vi "Teleop.vi"(10 "Match Info":T1={"Autonomous Elapsed Seconds"=0.0, "TeleOp Elapsed Seconds"=0.0, "Disabled Elapsed Seconds"=0.0, "Visited Autonomous"=FALSE, "Visited TeleOp"=FALSE, "Visited Disabled"=FALSE, "Autonomous Settings"={"Autonomous Style"=enum."Independent", "VI Refnum"=refnum}}, 11 "Call Context":T2) -> ()   [LabVIEW 2020]
doc: "This VI is called for each TeleOp packet received from the DS where the robot is not disabled. It is often used to read from the joysticks and update I/O or to update setpoints for timed control loops. It should complete and return within 20 milliseconds or it may miss DS packets."
uses:
  <vilib>/Rock Robotics/WPI/DriverStation/WPI_DriverStationDerivedRobotMode.ctl
  <vilib>/Rock Robotics/WPI/DriverStation/WPI_DriverStationMatch Info.ctl
  <vilib>/Rock Robotics/WPI/Solenoid/WPI_SolenoidValue.ctl
  <vilib>/Rock Robotics/WPI/ThirdParty/Phoenix-LabVIEW/Motor Controller/Controls/CTRE_Phoenix_MotorControl_ControlMode.ctl
  <vilib>/Rock Robotics/WPI/Utilities/WPI_GetSetVariantRefNum.vi
  <vilib>/Rock Robotics/Network Tables/NT Write Boolean Array.vi
  <vilib>/Rock Robotics/Network Tables/NT Write Numeric Array.vi
  <vilib>/Rock Robotics/Network Tables/NT Read Boolean.vi
  <vilib>/Rock Robotics/Network Tables/NT Read Number.vi
  <vilib>/Rock Robotics/WPI/Solenoid/Deprecated/WPI_SolenoidSetBool.vi
  <vilib>/Rock Robotics/Network Tables/NT Write Number.vi
  <vilib>/Rock Robotics/WPI/Solenoid/WPI_SolenoidSetEnum.vi
  Robot Global Data.vi
  <vilib>/Rock Robotics/WPI/Solenoid/Deprecated/WPI_SolenoidGetBool.vi
panel:
  out "TargetValid 5":bool
  out "TargetValid 4":bool
  out "POVs":i16[](array[numeric])
  out "Sample Slider 0":dbl(slide) scale=0.0..5.0
  out "Sample Boolean 1":bool
  out "Sample Boolean 0":bool
  # "April tags"
  # "Retroreflective tape"
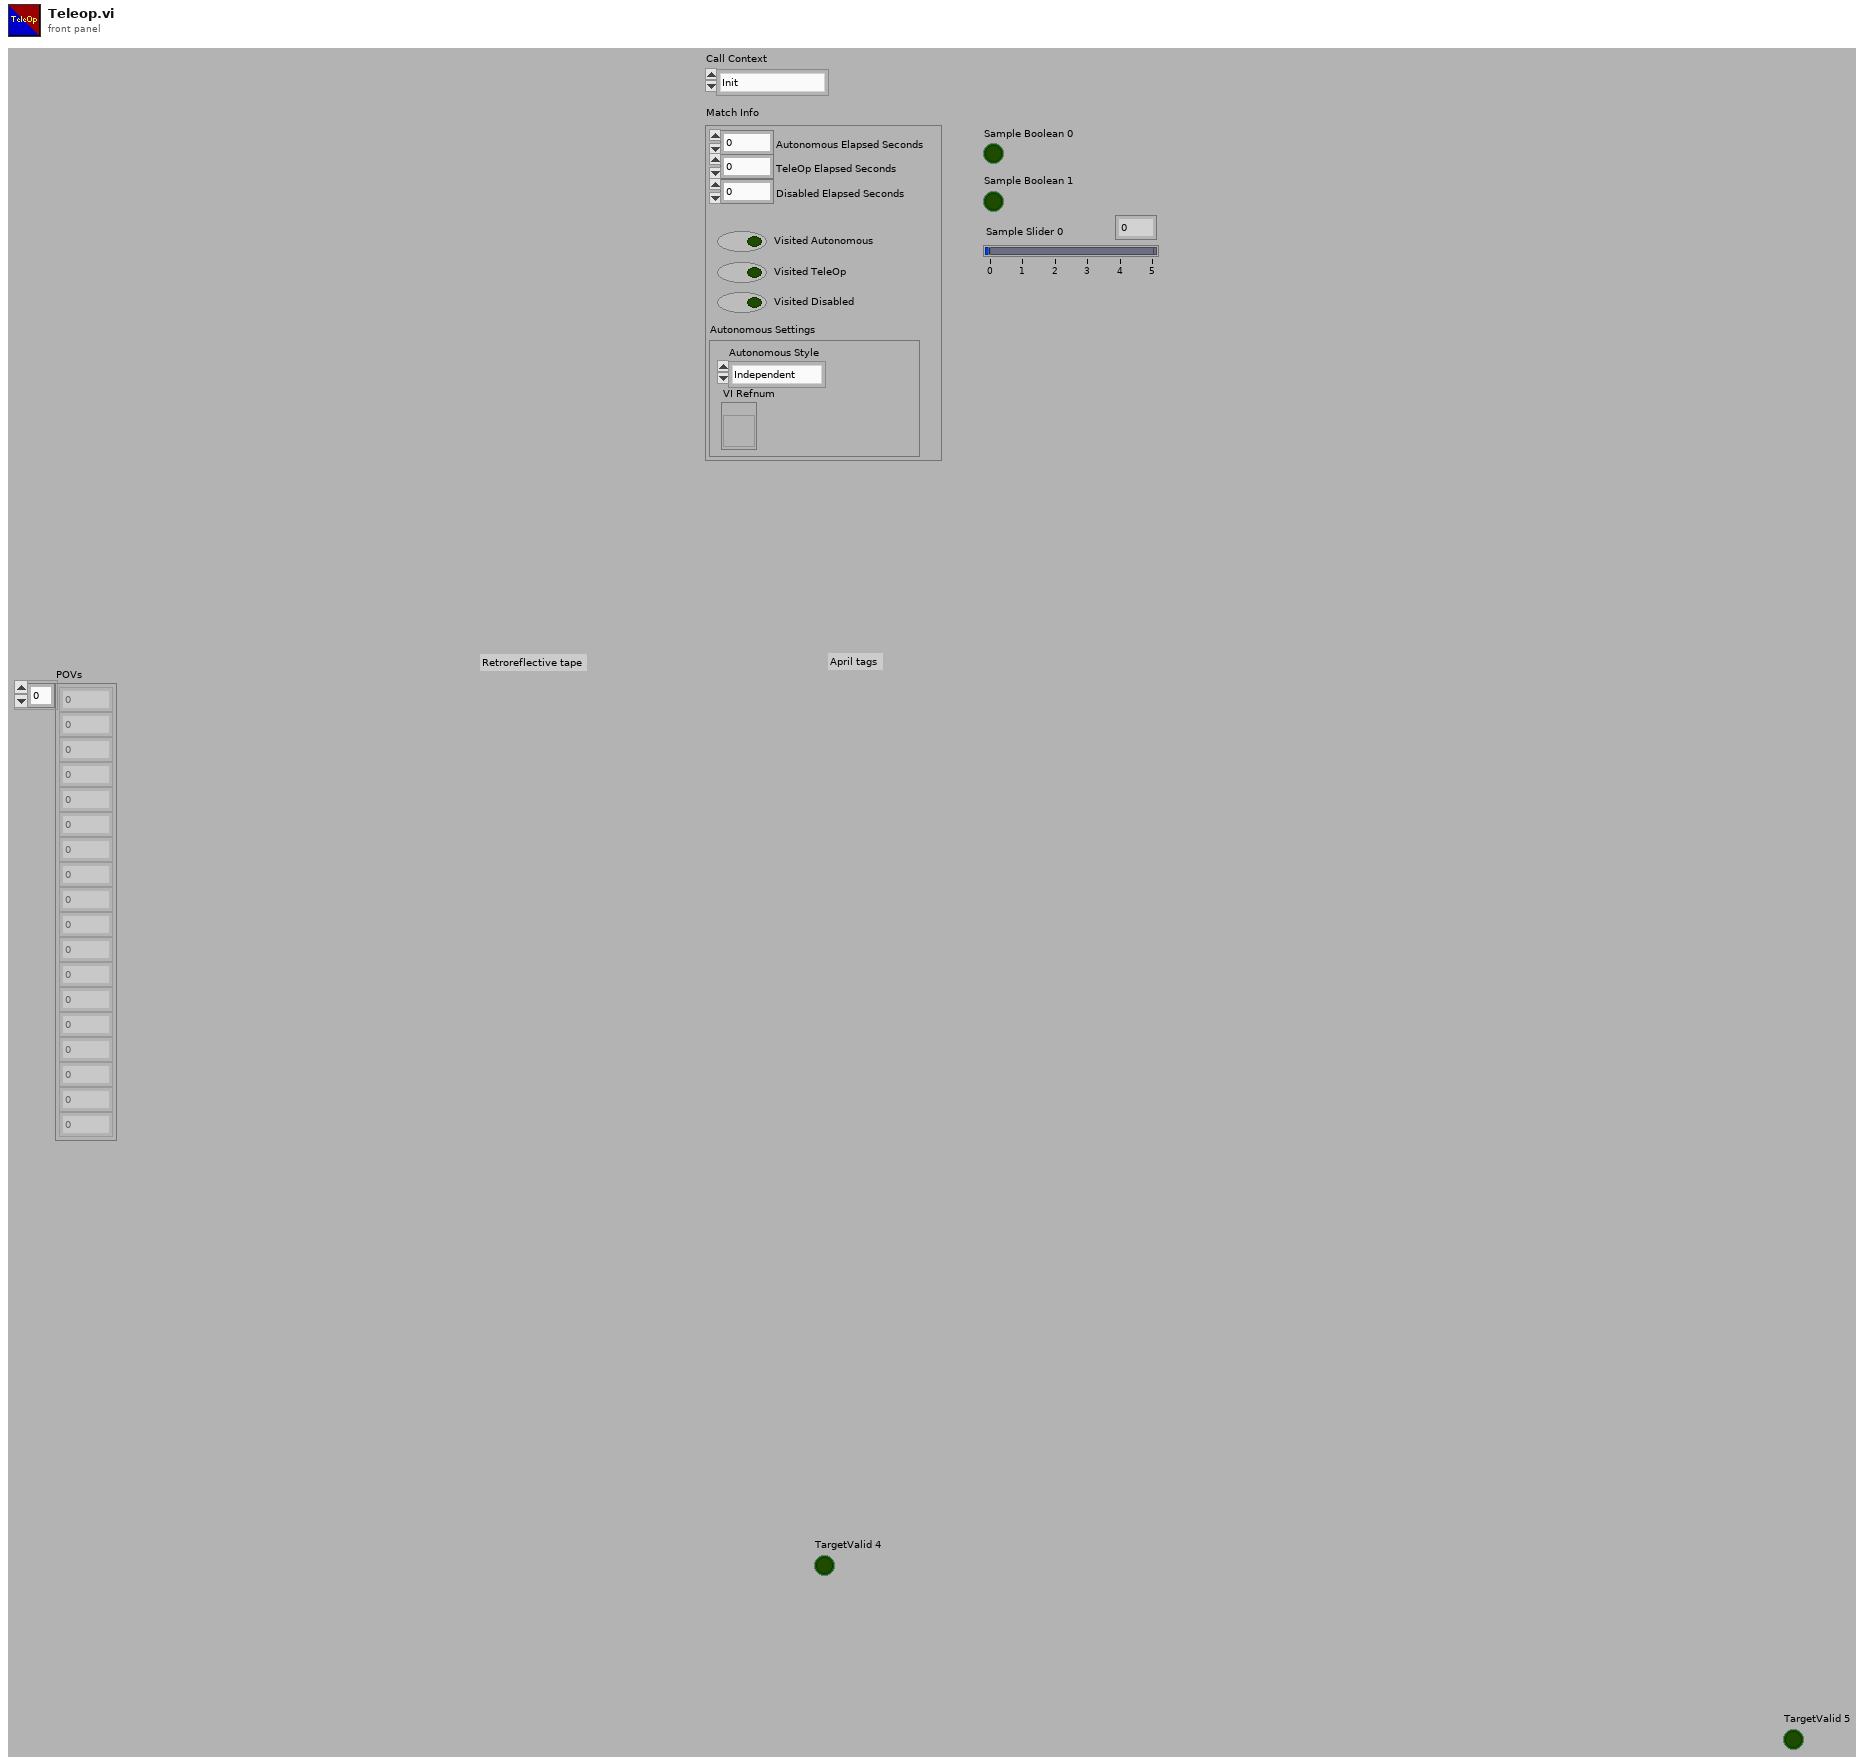
[diagram p1: front panel]
types:
  T1 = typedef "WPI_DriverStationMatch Info.ctl" = cluster{"Autonomous Elapsed Seconds":dbl, "TeleOp Elapsed Seconds":dbl, "Disabled Elapsed Seconds":dbl, "Visited Autonomous":bool, "Visited TeleOp":bool, "Visited Disabled":bool, "Autonomous Settings":cluster{"Autonomous Style":enum16{"Iterative", "Independent"}, "VI Refnum":refnum<vi>}}
  T2 = typedef "WPI_DriverStationDerivedRobotMode.ctl" = enum16{"Init", "Execute", "Stop"}
  T3 = typedef "WPI_SolenoidValue.ctl" = enum16{"Off", "On", "Forward", "Reverse"}
  T4 = cluster{"offsetAngle H":dbl, "offsetAngle V":dbl, "area":dbl, "skew":dbl}
  T5 = typedef "WPI_JoystickDevRef.ctl" = cluster{"Device":T6}
  T6 = typedef "WPI_JoystickDeviceEnum.ctl" = enum16{"USB 0", "USB 1", "USB 2", "USB 3", "USB 4", "USB 5"}
  T7 = cluster{"Buttons[0]":bool, "Buttons[1]":bool, "Buttons[2]":bool, "Buttons[3]":bool, "Buttons[4]":bool, "Buttons[5]":bool, "Buttons[6]":bool, "Buttons[7]":bool, "Buttons[8]":bool}
  T8 = cluster{"Axes[0]":dbl, "Axes[1]":dbl, "Axes[2]":dbl, "Axes[3]":dbl, "Axes[4]":dbl, "Axes[5]":dbl, "Axes[6]":dbl, "Axes[7]":dbl, "Axes[8]":dbl}
  T9 = typedef "WPI_RobotDriveDevRef.ctl" = cluster{"DevStatus":errorcluster, "Motors[]":T10[], "Square Inputs":bool, "Max Output":dbl}
  T10 = typedef "WPI_MotorControlDeviceRef.ctl" = cluster{"DeviceStatus":errorcluster, "Type":T11, "PWM":cluster{"PWM Channel":T12, "DeadBand":T13}, "CAN":cluster{"Device Number":u8, "SetOutput VI Ref":variant, "GetOutput VI Ref":variant, "Enable VI Ref":variant, "Disable VI Ref":variant, "Data":variant}, "Invert":bool, "DIO PWM":cluster{"PWM \"Enable\" Channel":T12, "DIOChannel":T14, "PWM Rate":dbl}}
  T11 = typedef "WPI_MotorControlType.ctl" = enum16{"PWM", "CAN", "DIO PWM"}
  T12 = typedef "FPGA_DIOPWMChannel.ctl" = enum8{"PWM 0", "PWM 1", "PWM 2", "PWM 3", "PWM 4", "PWM 5", "PWM 6", "PWM 7", "PWM 8", "PWM 9", "PWM MXP 0", "PWM MXP 1", "PWM MXP 2", "PWM MXP 3", "PWM MXP 4", "PWM MXP 5", "PWM MXP 6", "PWM MXP 7", "PWM MXP 8", "PWM MXP 9", "Invalid"}
  T13 = typedef "WPI_PWMDeadband.ctl" = cluster{"Name":string, "maxPositivePwm":i32, "minPositivePwm":i32, "centerPwm":i32, "maxNegativePwm":i32, "minNegativePwm":i32, "angularRange":u16}
  T14 = typedef "FPGA_DIOChannel.ctl" = enum8{"DIO 0", "DIO 1", "DIO 2", "DIO 3", "DIO 4", "DIO 5", "DIO 6", "DIO 7", "DIO 8", "DIO 9", "DIO MXP 0", "DIO MXP 1", "DIO MXP 2", "DIO MXP 3", "DIO MXP 4", "DIO MXP 5", "DIO MXP 6", "DIO MXP 7", "DIO MXP 8", "DIO MXP 9", "DIO MXP 10", "DIO MXP 11", "DIO MXP 12", "DIO MXP 13", "DIO MXP 14", "DIO MXP 15", "SPI Port CS1", "SPI Port CS2", "SPI Port CS3", "SPI Port MISO", "SPI Port MOSI", "Invalid"}
  T15 = typedef "WPI_SolenoidDevRef.ctl" = cluster{"DevStatus":errorcluster, "Pneumatics Control Module":u8, "Forward Solenoid Channel":T16, "Reverse Solenoid Channel":T16}
  T16 = typedef "WPI_SolenoidChannel.ctl" = enum8{"Solenoid 0", "Solenoid 1", "Solenoid 2", "Solenoid 3", "Solenoid 4", "Solenoid 5", "Solenoid 6", "Solenoid 7", "Solenoid 8", "Solenoid 9", "Solenoid 10", "Solenoid 11", "Solenoid 12", "Solenoid 13", "Solenoid 14", "Solenoid 15", "Invalid"}
  T17 = typedef "CTRE_Phoenix_MotorControl_ControlMode.ctl" = u16
  T18 = cluster{"Motors[][0]":T10, "Motors[][1]":T10, "Motors[][2]":T10, "Motors[][3]":T10, "Motors[][4]":T10, "Motors[][5]":T10, "Motors[][6]":T10, "Motors[][7]":T10, "Motors[][8]":T10}
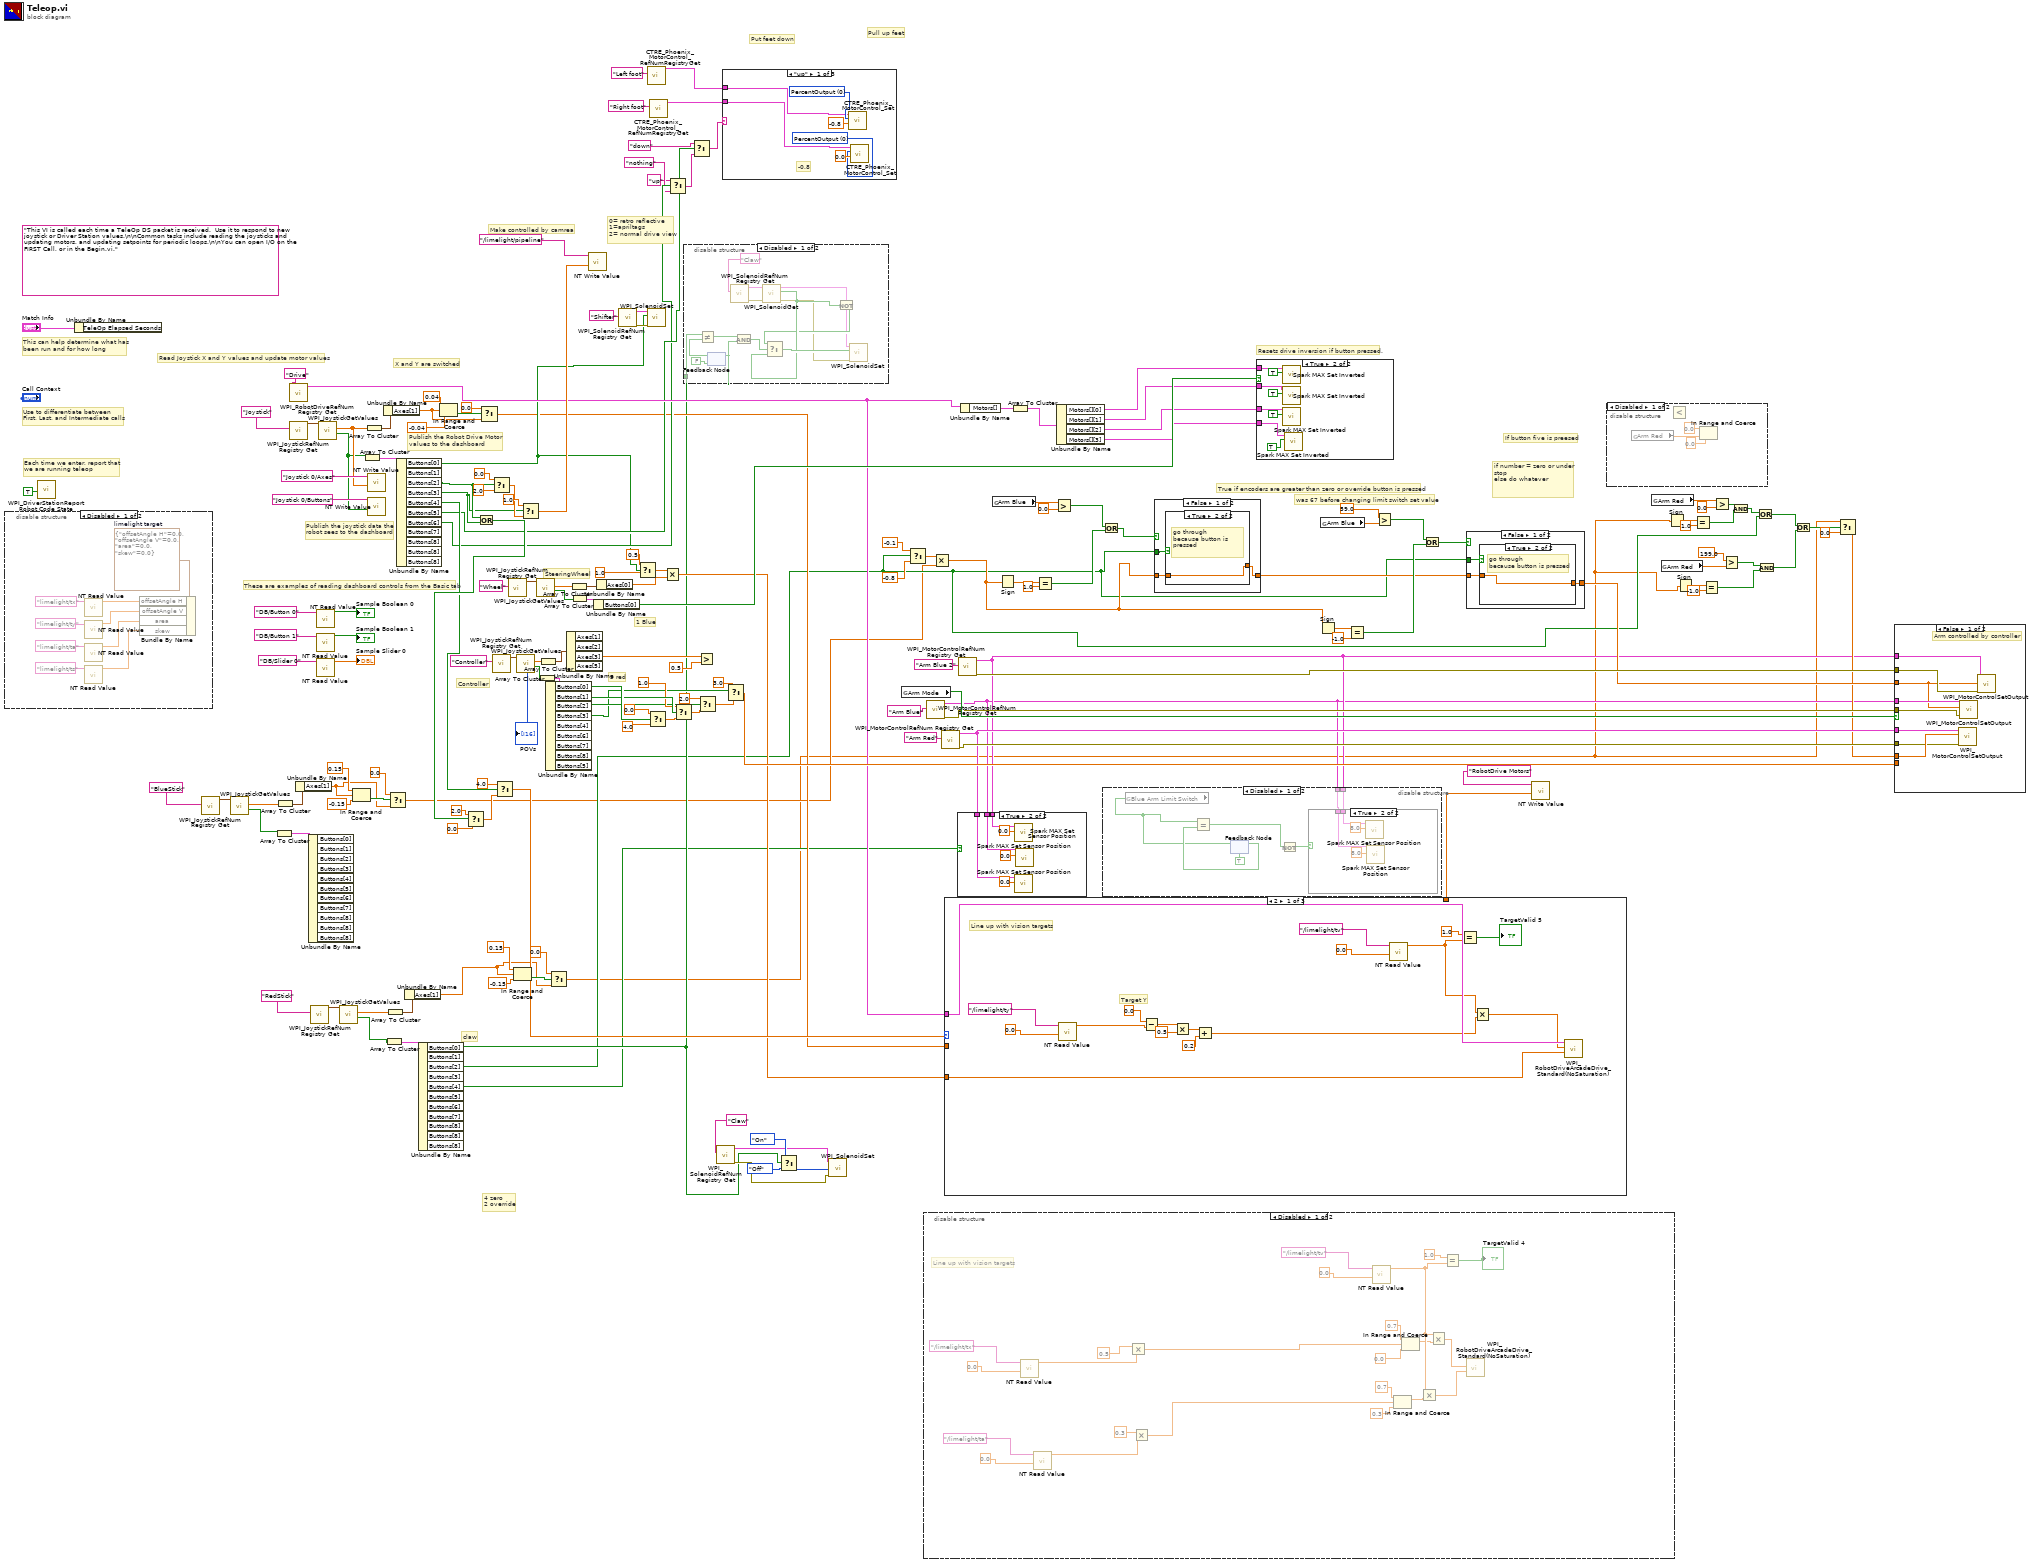
[diagram p0: block diagram]
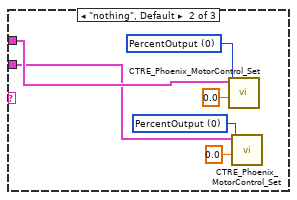
[diagram p6: hidden frame]
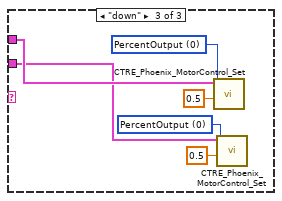
[diagram p7: hidden frame]
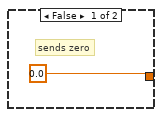
[diagram p8: hidden frame]
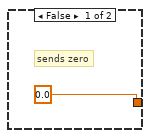
[diagram p10: hidden frame]
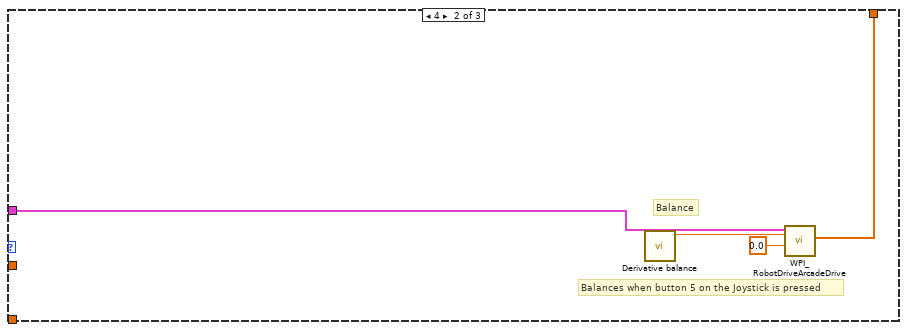
[diagram p15: hidden frame]
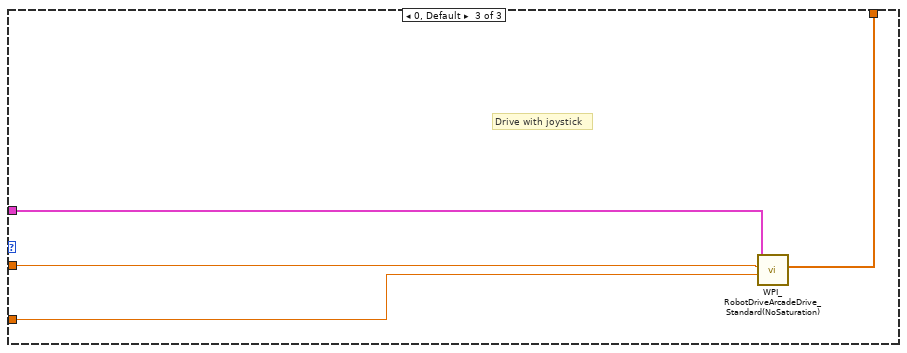
[diagram p16: hidden frame]
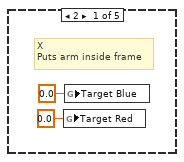
[diagram p18: hidden frame]
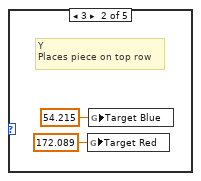
[diagram p19: hidden frame]
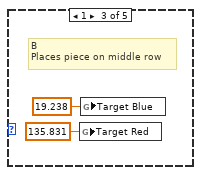
[diagram p20: hidden frame]
diagram:
  (unwired) "This VI is called each time a TeleOp DS packet is received.  Use it to respond to new joystick or Driver Station values.\n\nCommon tasks include reading the joysticks and updating motors, and updating setpoints for periodic loops.\n\nYou can open I/O on the FIRST Call, or in the Begin.vi."
  # "4 zero\n2 override"
  # "claw"
  # "5 red"
  # "1 Blue"
  # "X and Y are switched"
  # "Put feet down"
  # "Pull up feet"
  # "was 67 before changing limit switch set value"
  # "True if encoders are greater than zero or override button is pressed"
  # "if number = zero or under\nstop\nelse do whatever"
  # "If button five is preesed"
  # "Resets drive inversion if button pressed."
  # "0= retro reflective\n1=apriltags\n2= normal drive view"
  # "Make controlled by camrea"
  # "SteeringWheel"
  # "Controller"
  # "These are examples of reading dashboard controls from the Basic tab"
  # "Publish the Robot Drive Motor\nvalues to the dashboard"
  # "Publish the joystick data the\nrobot sees to the dashboard"
  # "Each time we enter, report that\nwe are running teleop"
  # "Use to differentiate between\nFirst, Last, and Intermediate calls"
  # "This can help determine what has\nbeen run and for how long"
  # "Read Joystick X and Y values and update motor values"
  n1 = disable-structure shown="Disabled" {
    frame Disabled {
      w182 = T4 {"offsetAngle H"=0.0, "offsetAngle V"=0.0, "area"=0.0, "skew"=0.0}  # limelight target
      n2 = call-poly <vilib>:"NT Read Value.vi"("name"="limelight/tx" ("Name")) -> ("value"=w181:dbl)  [unwired: 8 in, 2 out]
      n3 = call-poly <vilib>:"NT Read Value.vi"("name"="limelight/ty" ("Name")) -> ("value"=w180:dbl)  [unwired: 8 in, 2 out]
      n4 = call-poly <vilib>:"NT Read Value.vi"("name"="limelight/ta" ("Name")) -> ("value"=w179:dbl)  [unwired: 8 in, 2 out]
      n5 = call-poly <vilib>:"NT Read Value.vi"("name"="limelight/ts" ("Name")) -> ("value"=w178:dbl)  [unwired: 8 in, 2 out]
      n6 = Bundle By Name(cluster=w182, "offsetAngle H"=w181, "offsetAngle V"=w180, "area"=w179, "skew"=w178) -> ()  [unwired: 1 out]
    }
    frame Enabled {
    }
  }
  n7 = call <vilib>:"WPI_DriverStationReport Robot Code State.vi"("TeleOp"=TRUE ("Autonomous")) -> ()  [unwired: 10 in, 1 out]
  n8 = Unbundle By Name("Match Info") -> ()  [unwired: 1 out]
  n9 = call <vilib>:"WPI_JoystickRefNum Registry Get.vi"("refnum name"="BlueStick") -> ("JoystickDevRef"=w26:T5)  [unwired: 1 in, 9 out]
  n10 = call <vilib>:"WPI_JoystickGetValues.vi"("JoystickDevRef"=w26) -> ("Buttons"=w23:bool[], "Axes"=w25:dbl[])  [unwired: 6 in, 3 out]
  n11 = Array To Cluster(array=w23) -> (cluster=w22:T7)
  n12 = Array To Cluster(array=w25) -> (cluster=w24:T8)
  n13 = call <vilib>:"WPI_RobotDriveRefNum Registry Get.vi"("refnum name"="Drive") -> ("RobotDriveDevRef"=w102:T9)  [unwired: 1 in, 9 out]
  n14 = call <vilib>:"WPI_JoystickRefNum Registry Get.vi"("refnum name"="Joystick") -> ("JoystickDevRef"=w174:T5)  [unwired: 1 in, 9 out]
  n15 = Unbundle By Name(w24) -> ("Axes[1]"=w8:dbl)
  n16 = Unbundle By Name(w22) -> ()  [unwired: 11 out]
  n17 = call <vilib>:"WPI_JoystickRefNum Registry Get.vi"("refnum name"="RedStick") -> ("JoystickDevRef"=w17:T5)  [unwired: 1 in, 9 out]
  n18 = call-poly <vilib>:"NT Read Value.vi"("name"="DB/Button 0" ("refnum name")) -> ("value"=→"Sample Boolean 0":bool)  [unwired: 8 in, 2 out]
  n19 = call-poly <vilib>:"NT Read Value.vi"("name"="DB/Slider 0" ("refnum name")) -> ("value"=→"Sample Slider 0":dbl)  [unwired: 8 in, 2 out]
  n20 = call-poly <vilib>:"NT Read Value.vi"("name"="DB/Button 1" ("refnum name")) -> ("value"=→"Sample Boolean 1":bool)  [unwired: 8 in, 2 out]
  n21 = call <vilib>:"WPI_JoystickGetValues.vi"("JoystickDevRef"=w174) -> ("Buttons"=w132:bool[], "Axes"=w163:dbl[])  [unwired: 6 in, 3 out]
  n22 = call <vilib>:"WPI_JoystickGetValues.vi"("JoystickDevRef"=w17) -> ("Buttons"=w20:bool[], "Axes"=w18:dbl[])  [unwired: 6 in, 3 out]
  n23 = In Range and Coerce(upper limit=0.15, x=w8, lower limit=-0.15) -> (In Range?=w10:bool)  [unwired: 1 out]
  n24 = Array To Cluster(array=w132) -> (cluster=w131:T7)
  n25 = Array To Cluster(array=w163) -> (cluster=w162:T8)
  n26 = call-poly <vilib>:"NT Write Value.vi"("value"=w163, "name"="Joystick 0/Axes" ("Name")) -> ()  [unwired: 9 in, 1 out]
  n27 = call-poly <vilib>:"NT Write Value.vi"("value"=w132, "name"="Joystick 0/Buttons" ("Name")) -> ()  [unwired: 9 in, 1 out]
  n28 = Unbundle By Name(w162) -> ("Axes[1]"=w33:dbl)
  n29 = Array To Cluster(array=w20) -> (cluster=w21:T7)
  n30 = Array To Cluster(array=w18) -> (cluster=w19:T8)
  n31 = Select(t=0.0, s=w10, f=w8) -> (s? t:f=w7:dbl)
  n32 = Unbundle By Name(w131) -> ("Buttons[0]"=w42:bool, "Buttons[2]"=w115:bool, "Buttons[3]"=w114:bool, "Buttons[4]"=w61:bool, "Buttons[5]"=w60:bool, "Buttons[6]"=w56:bool)  [unwired: 5 out]
  n33 = Unbundle By Name(w19) -> ("Axes[1]"=w2:dbl)
  n34 = Unbundle By Name(w21) -> ("Buttons[0]"=w15:bool, "Buttons[2]"=w13:bool, "Buttons[4]"=w14:bool)  [unwired: 8 out]
  n35 = In Range and Coerce(upper limit=0.04, x=w33, lower limit=-0.04) -> (In Range?=w37:bool)  [unwired: 1 out]
  n36 = Or(x=w115, y=w114) -> (x .or. y?=w113:bool)
  n37 = Select(t=2.0, s=w113, f=0.0) -> (s? t:f=w128:dbl)
  n38 = Select(t=0.0, s=w37, f=w33) -> (s? t:f=w32:dbl)
  n39 = Select(t=0.0, s=w115, f=2.0) -> (s? t:f=w116:dbl)
  n40 = call <vilib>:"WPI_JoystickRefNum Registry Get.vi"("refnum name"="Controller") -> ("JoystickDevRef"=w156:T5)  [unwired: 9 in, 1 out]
  n41 = Select(t=4.0, s=w61, f=w128) -> (s? t:f=w126:dbl)
  n42 = call <vilib>:"WPI_JoystickRefNum Registry Get.vi"("refnum name"="Wheel") -> ("JoystickDevRef"=w160:T5)  [unwired: 9 in, 1 out]
  n43 = In Range and Coerce(upper limit=0.15, x=w2, lower limit=-0.15) -> (In Range?=w4:bool)  [unwired: 1 out]
  n44 = call <vilib>:"WPI_JoystickGetValues.vi"("JoystickDevRef"=w156) -> ("Buttons"=w153:bool[], "Axes"=w155:dbl[], "POVs"=→"POVs":i16[])  [unwired: 6 in, 2 out]
  n45 = Select(t=1.0, s=w114, f=w116) -> (s? t:f=w111:dbl)
  n46 = call <vilib>:"WPI_JoystickGetValues.vi"("JoystickDevRef"=w160) -> ("Buttons"=w107:bool[], "Axes"=w159:dbl[])  [unwired: 6 in, 3 out]
  n47 = Array To Cluster(array=w153) -> (cluster=w152:T7)
  n48 = Array To Cluster(array=w155) -> (cluster=w154:T8)
  n49 = Unbundle By Name(w152) -> ("Buttons[0]"=w150:bool, "Buttons[1]"=w145:bool, "Buttons[2]"=w138:bool, "Buttons[3]"=w137:bool)  [unwired: 5 out]
  n50 = Select(t=0.0, s=w4, f=w2) -> (s? t:f=w1:dbl)
  n51 = Unbundle By Name(w154) -> ("Axes[3]"=w120:dbl)  [unwired: 3 out]
  n52 = Array To Cluster(array=w159) -> (cluster=w158:T8)
  n53 = Array To Cluster(array=w107) -> (cluster=w106:T7)
  n54 = call-poly <vilib>:"NT Write Value.vi"("value"=w111, "name"="/limelight/pipeline" ("Name")) -> ()  [unwired: 9 in, 1 out]
  n55 = Unbundle By Name(w106) -> ("Buttons[0]"=w105:bool)
  n56 = Unbundle By Name(w158) -> ("Axes[0]"=w41:dbl)
  n57 = call <vilib>:"WPI_SolenoidRefNum Registry Get.vi"("refnum name"="Shifter") -> ("error out"=w124:errorcluster, "SolenoidDevRef"=w123:T15)  [unwired: 9 in]
  n58 = Select(t=0.5, s=w42, f=1.0) -> (s? t:f=w43:dbl)
  n59 = call <vilib>:"CTRE_Phoenix_MotorControl_RefNumRegistryGet.vi"("refnum name"="Left foot") -> ("PhoenixMotorControlDevRef"=w50:T10)  [unwired: 9 in, 1 out]
  n60 = call-poly <vilib>:"WPI_SolenoidSet.vi"("error in (no error)"=w124, "Value"=w42, "SolenoidDevRef"=w123) -> ()  [unwired: 7 in, 2 out]
  n61 = call <vilib>:"CTRE_Phoenix_MotorControl_RefNumRegistryGet.vi"("refnum name"="Right foot") -> ("PhoenixMotorControlDevRef"=w51:T10)  [unwired: 9 in, 1 out]
  n62 = Select(t=0.0, s=w150, f=4.0) -> (s? t:f=w147:dbl)
  n63 = Multiply(x=w43, y=w41) -> (x*y=w40:dbl)
  n64 = Select(t="up", s=w56, f="nothing") -> (s? t:f=w57:string)
  n65 = Select(t=1.0, s=w145, f=w147) -> (s? t:f=w146:dbl)
  n66 = disable-structure shown="Disabled" {
    disable-tunnel: w15 -> [w194 _]
    frame Disabled {
      n67 = feedback #1(FALSE ("x > y?")) -> (w198:bool)
      n68 = Not Equal?(x=w194, y=w198) -> (x != y?=w196:bool)
      n69 = feedback-in #1(w194) -> ()
      n70 = call <vilib>:"WPI_SolenoidRefNum Registry Get.vi"("refnum name"="Claw") -> ("error out"=w192:errorcluster, "SolenoidDevRef"=w193:T15)  [unwired: 9 in]
      n71 = And(x=w196, y=w194) -> (x .and. y?=w195:bool)
      n72 = call-poly <vilib>:"WPI_SolenoidGet.vi"("error in (no error)"=w192, "SolenoidDevRef"=w193) -> ("error out"=w187:errorcluster, "Value"=w190:bool, "SolenoidDevRef"=w188:T15)  [unwired: 7 in]
      n73 = Not(x=w190) -> (.not. x?=w189:bool)
      n74 = Select(t=w189, s=w195, f=w190) -> (s? t:f=w199:bool)
      n75 = call-poly <vilib>:"WPI_SolenoidSet.vi"("error in (no error)"=w187, "Value"=w199, "SolenoidDevRef"=w188) -> ()  [unwired: 7 in, 2 out]
    }
    frame Enabled {
    }
  }
  n76 = Select(t="down", s=w60, f=w57) -> (s? t:f=w58:string)
  n77 = Greater?(x=w120, y=0.5) -> ()  [unwired: 1 out]
  n78 = Select(t=2.0, s=w138, f=w146) -> (s? t:f=w135:dbl)
  n79 = call <vilib>:"WPI_SolenoidRefNum Registry Get.vi"("refnum name"="Claw") -> ("error out"=w44:errorcluster, "SolenoidDevRef"=w45:T15)  [unwired: 9 in]
  n80 = case shown="\"up\"" w58 {
    tunnel: w51 -> [w201 w206 w212]
    tunnel: w50 -> [w200 w207 w213]
    frame "up" {
      w204 = T17 0 items=["PercentOutput"=0, "Position"=1, "Velocity"=2, "Current"=3, "Follower"=5, "MotionProfile"=6, "MotionMagic"=7, "MotionProfileArc"=10, "Disabled"=15] ("Control Mode")
      w202 = T17 0 items=["PercentOutput"=0, "Position"=1, "Velocity"=2, "Current"=3, "Follower"=5, "MotionProfile"=6, "MotionMagic"=7, "MotionProfileArc"=10, "Disabled"=15] ("Control Mode")
      # "-0.8"
      n81 = call <vilib>:"CTRE_Phoenix_MotorControl_Set.vi"("Output"=-0.8, "Control Mode"=w202, "PhoenixMotorControlDevRef"=w200) -> ()  [unwired: 7 in, 2 out]
      n82 = call <vilib>:"CTRE_Phoenix_MotorControl_Set.vi"("Output"=0.0, "Control Mode"=w204, "PhoenixMotorControlDevRef"=w201) -> ()  [unwired: 7 in, 2 out]
    }
    frame "nothing", Default {
      w209 = T17 0 items=["PercentOutput"=0, "Position"=1, "Velocity"=2, "Current"=3, "Follower"=5, "MotionProfile"=6, "MotionMagic"=7, "MotionProfileArc"=10, "Disabled"=15] ("Control Mode")
      w211 = T17 0 items=["PercentOutput"=0, "Position"=1, "Velocity"=2, "Current"=3, "Follower"=5, "MotionProfile"=6, "MotionMagic"=7, "MotionProfileArc"=10, "Disabled"=15] ("Control Mode")
      n83 = call <vilib>:"CTRE_Phoenix_MotorControl_Set.vi"("Output"=0.0, "Control Mode"=w211, "PhoenixMotorControlDevRef"=w207) -> ()  [unwired: 7 in, 2 out]
      n84 = call <vilib>:"CTRE_Phoenix_MotorControl_Set.vi"("Output"=0.0, "Control Mode"=w209, "PhoenixMotorControlDevRef"=w206) -> ()  [unwired: 7 in, 2 out]
    }
    frame "down" {
      w215 = T17 0 items=["PercentOutput"=0, "Position"=1, "Velocity"=2, "Current"=3, "Follower"=5, "MotionProfile"=6, "MotionMagic"=7, "MotionProfileArc"=10, "Disabled"=15] ("Control Mode")
      w217 = T17 0 items=["PercentOutput"=0, "Position"=1, "Velocity"=2, "Current"=3, "Follower"=5, "MotionProfile"=6, "MotionMagic"=7, "MotionProfileArc"=10, "Disabled"=15] ("Control Mode")
      n85 = call <vilib>:"CTRE_Phoenix_MotorControl_Set.vi"("Output"=0.5, "Control Mode"=w217, "PhoenixMotorControlDevRef"=w213) -> ()  [unwired: 7 in, 2 out]
      n86 = call <vilib>:"CTRE_Phoenix_MotorControl_Set.vi"("Output"=0.5, "Control Mode"=w215, "PhoenixMotorControlDevRef"=w212) -> ()  [unwired: 7 in, 2 out]
    }
  }
  n87 = Select(t=3.0, s=w137, f=w135) -> (s? t:f=w134:dbl)
  n88 = Select(t=WPI_SolenoidValue."On" ("Value"), s=w15, f=WPI_SolenoidValue."Off" ("Value")) -> (s? t:f=w48:T3)
  n89 = call-poly <vilib>:"WPI_SolenoidSet.vi"("error in (no error)"=w44, "Value"=w48, "SolenoidDevRef"=w45) -> ()  [unwired: 7 in, 2 out]
  n90 = global read "Robot Global Data.vi" "Arm Mode"() -> (w151:bool)
  n91 = Select(t=-0.1, s=w13, f=-0.8) -> (s? t:f=w31:dbl)
  n92 = disable-structure shown="Disabled" {
    frame Disabled {
      # "Line up with vision targets"
      n93 = call-poly <vilib>:"NT Read Value.vi"("default value"=0.0 ("Default Value"), "name"="/limelight/tx" ("Name")) -> ("value"=w219:dbl)  [unwired: 7 in, 2 out]
      n94 = call-poly <vilib>:"NT Read Value.vi"("default value"=0.0 ("Default Value"), "name"="/limelight/ta" ("Name")) -> ("value"=w223:dbl)  [unwired: 7 in, 2 out]
      n95 = Multiply(x=0.5, y=w219) -> (x*y=w218:dbl)
      n96 = Multiply(x=0.3, y=w223) -> (x*y=w222:dbl)
      n97 = call-poly <vilib>:"NT Read Value.vi"("default value"=0.0 ("Default Value"), "name"="/limelight/tv" ("Name")) -> ("value"=w230:dbl)  [unwired: 7 in, 2 out]
      n98 = In Range and Coerce(upper limit=0.7, x=w222, lower limit=0.3) -> (coerced(x)=w229:dbl)  [unwired: 1 out]
      n99 = In Range and Coerce(upper limit=0.7, x=w218, lower limit=0.0) -> (coerced(x)=w228:dbl)  [unwired: 1 out]
      n100 = Multiply(x=w230, y=w229) -> (x*y=w232:dbl)
      n101 = Multiply(x=w230, y=w228) -> (x*y=w231:dbl)
      n102 = Equal?(x=1.0, y=w230) -> (x = y?=→"TargetValid 4":bool)
      n103 = call <vilib>:"WPI_RobotDriveArcadeDrive_Standard(NoSaturation).vi"("Y axis value"=w232, "X axis value"=w231) -> ()  [unwired: 2 in, 8 out]
    }
    frame Enabled {
    }
  }
  n104 = call <vilib>:"WPI_MotorControlRefNum Registry Get.vi"("refnum name"="Arm Blue") -> ("error out"=w141:errorcluster, "MotorControlDevRef"=w62:T10)  [unwired: 9 in]
  n105 = Multiply(x=w31, y=w7) -> (x*y=w28:dbl)
  n106 = call <vilib>:"WPI_MotorControlRefNum Registry Get.vi"("refnum name"="Arm Red") -> ("error out"=w139:errorcluster, "MotorControlDevRef"=w108:T10)  [unwired: 9 in]
  n107 = case shown="2" w126 {
    tunnel: w102 -> [w255 w261 w265]
    tunnel: w32 -> [_ _ w264]
    tunnel: w40 -> [w241 _ w263]
    tunnel: [_ w260 w262] -> w125
    frame 2 {
      # "Target Y"
      # "Line up with vision targets"
      n108 = call-poly <vilib>:"NT Read Value.vi"("default value"=0.0 ("Default Value"), "name"="/limelight/ty" ("Name")) -> ("value"=w245:dbl)  [unwired: 7 in, 2 out]
      n109 = Subtract(x=0.0, y=w245) -> (x-y=w254:dbl)
      n110 = Multiply(x=w254, y=0.5) -> (x*y=w246:dbl)
      n111 = Add(x=w246, y=0.2) -> (x+y=w242:dbl)
      n112 = call-poly <vilib>:"NT Read Value.vi"("default value"=0.0 ("Default Value"), "name"="/limelight/tv" ("Name")) -> ("value"=w249:dbl)  [unwired: 7 in, 2 out]
      n113 = Equal?(x=1.0, y=w249) -> (x = y?=→"TargetValid 5":bool)
      n114 = Multiply(x=w249, y=w242) -> (x*y=w248:dbl)
      n115 = call <vilib>:"WPI_RobotDriveArcadeDrive_Standard(NoSaturation).vi"("Y axis value"=w241, "X axis value"=w248, "RobotDriveDevRef"=w255) -> ()  [unwired: 1 in, 8 out]
    }
    frame 4 {
      # "Balances when button 5 on the Joystick is pressed"
      # "Balance"
      n116 = call "Derivative balance.vi"() -> ("Motor Power"=w259:dbl)  [unwired: 11 in]
      n117 = call-poly <vilib>:"WPI_RobotDriveArcadeDrive.vi"("Y axis value"=0.0, "X axis value"=w259, "RobotDriveDevRef"=w261) -> ("Motor Values"=w260:dbl[])  [unwired: 6 in, 2 out]
    }
    frame 0, Default {
      # "Drive with joystick"
      n118 = call <vilib>:"WPI_RobotDriveArcadeDrive_Standard(NoSaturation).vi"("Y axis value"=w263, "X axis value"=w264, "RobotDriveDevRef"=w265) -> ("Motor Values"=w262:dbl[])  [unwired: 1 in, 7 out]
    }
  }
  n119 = call <vilib>:"WPI_MotorControlRefNum Registry Get.vi"("refnum name"="Arm Blue 2") -> ("error out"=w109:errorcluster, "MotorControlDevRef"=w63:T10)  [unwired: 9 in]
  n120 = case shown="True" w14 {
    tunnel: w63 -> [_ w271]
    tunnel: w62 -> [_ w270]
    tunnel: w108 -> [_ w269]
    frame False {
    }
    frame True {
      n121 = call <vilib>:"Spark MAX Set Sensor Position.vi"("Position"=0.0, "MotorControlDeviceRef"=w271) -> ()  [unwired: 8 in, 2 out]
      n122 = call <vilib>:"Spark MAX Set Sensor Position.vi"("Position"=0.0, "MotorControlDeviceRef"=w269) -> ()  [unwired: 8 in, 2 out]
      n123 = call <vilib>:"Spark MAX Set Sensor Position.vi"("Position"=0.0, "MotorControlDeviceRef"=w270) -> ()  [unwired: 8 in, 2 out]
    }
  }
  n124 = Unbundle By Name(w102) -> ("Motors[]"=w104:T10[])
  n125 = global read "Robot Global Data.vi" "Arm Blue"() -> (w97:dbl)
  n126 = Sign(1:w28) -> (0:w94:dbl)
  n127 = Array To Cluster(array=w104) -> (cluster=w103:T18)
  n128 = Equal?(x=w94, y=1.0) -> (x = y?=w92:bool)
  n129 = Greater?(x=w97, y=0.0) -> (0:w96:bool)
  n130 = Unbundle By Name(w103) -> ("Motors[][0]"=w101:T10, "Motors[][1]"=w99:T10, "Motors[][2]"=w98:T10, "Motors[][3]"=w100:T10)
  n131 = Or(x=w96, y=w92) -> (x .or. y?=w91:bool)
  n132 = disable-structure shown="Disabled" {
    disable-tunnel: w63 -> [w277 _]
    disable-tunnel: w62 -> [w276 _]
    frame Disabled {
      n133 = global read "Robot Global Data.vi" "Blue Arm Limit Switch"() -> (w273:bool)
      n134 = feedback #2(TRUE) -> (w274:bool)
      n135 = Equal?(x=w273, y=w274) -> (x = y?=w272:bool)
      n136 = feedback-in #2(w273) -> ()
      n137 = Not(x=w272) -> (.not. x?=w278:bool)
      n138 = case shown="True" w278 {
        tunnel: w277 -> [_ w282]
        tunnel: w276 -> [_ w281]
        frame False {
        }
        frame True {
          n139 = call <vilib>:"Spark MAX Set Sensor Position.vi"("Position"=8.0, "MotorControlDeviceRef"=w282) -> ()  [unwired: 8 in, 2 out]
          n140 = call <vilib>:"Spark MAX Set Sensor Position.vi"("Position"=8.0, "MotorControlDeviceRef"=w281) -> ()  [unwired: 8 in, 2 out]
        }
      }
    }
    frame Enabled {
    }
  }
  n141 = case shown="False" w91 {
    tunnel: w13 -> [w285 _]
    tunnel: [w284 w288] -> w83
    tunnel: w28 -> [w283 w288]
    frame False {
      n142 = case shown="True" w285 {
        tunnel: [0.0 w287] -> w284
        tunnel: w283 -> [_ w287]
        frame False {
          # "sends zero"
        }
        frame True {
          # "go through\nbecause button is pressed"
        }
      }
    }
    frame True {
      # "go through if\nin range or moveing in right derection"
    }
  }
  n143 = case shown="True" w105 {
    tunnel: w101 -> [_ w296]
    tunnel: w100 -> [_ w291]
    tunnel: w99 -> [_ w290]
    tunnel: w98 -> [_ w289]
    frame False {
    }
    frame True {
      n144 = call <vilib>:"Spark MAX Set Inverted.vi"("Inverted (F)"=TRUE, "MotorControlDeviceRef in"=w296) -> ()  [unwired: 8 in, 2 out]
      n145 = call <vilib>:"Spark MAX Set Inverted.vi"("Inverted (F)"=TRUE, "MotorControlDeviceRef in"=w290) -> ()  [unwired: 8 in, 2 out]
      n146 = call <vilib>:"Spark MAX Set Inverted.vi"("Inverted (F)"=TRUE, "MotorControlDeviceRef in"=w289) -> ()  [unwired: 8 in, 2 out]
      n147 = call <vilib>:"Spark MAX Set Inverted.vi"("Inverted (F)"=TRUE, "MotorControlDeviceRef in"=w291) -> ()  [unwired: 8 in, 2 out]
    }
  }
  n148 = Sign(1:w28) -> (0:w89:dbl)
  n149 = global read "Robot Global Data.vi" "Arm Blue"() -> (w85:dbl)
  n150 = Equal?(x=w89, y=-1.0) -> (x = y?=w87:bool)
  n151 = Greater?(x=59.0 ("y"), y=w85) -> (0:w90:bool)
  n152 = Or(x=w90, y=w87) -> (x .or. y?=w86:bool)
  n153 = case shown="False" w86 {
    tunnel: w13 -> [w299 _]
    tunnel: [w298 w302] -> w82
    tunnel: w83 -> [w297 w302]
    frame False {
      n154 = case shown="True" w299 {
        tunnel: [0.0 w301] -> w298
        tunnel: w297 -> [_ w301]
        frame False {
          # "sends zero"
        }
        frame True {
          # "go through\nbecause button is pressed"
        }
      }
    }
    frame True {
      # "go through if\nin range or moveing in right derection"
    }
  }
  n155 = call-poly <vilib>:"NT Write Value.vi"("value"=w125, "name"="RobotDrive Motors" ("Name")) -> ()  [unwired: 9 in, 1 out]
  n156 = disable-structure shown="Disabled" {
    frame Disabled {
      n157 = global read "Robot Global Data.vi" "Arm Red"() -> (w303:dbl)
      n158 = Less?() -> ()  [unwired: 2 in, 1 out]
      n159 = In Range and Coerce(upper limit=0.0, x=w303, lower limit=0.0) -> ()  [unwired: 2 out]
    }
    frame Enabled {
    }
  }
  n160 = global read "Robot Global Data.vi" "Arm Red"() -> (w81:dbl)
  n161 = global read "Robot Global Data.vi" "Arm Red"() -> (w75:dbl)
  n162 = Sign(1:w1) -> (0:w79:dbl)
  n163 = Sign(1:w1) -> (0:w77:dbl)
  n164 = Equal?(x=w79, y=1.0) -> (x = y?=w72:bool)
  n165 = Equal?(x=w77, y=-1.0) -> (x = y?=w71:bool)
  n166 = Greater?(x=w81, y=0.0) -> (0:w73:bool)
  n167 = Greater?(x=199.0 ("y"), y=w75) -> (0:w70:bool)
  n168 = And(x=w73, y=w72) -> (x .and. y?=w69:bool)
  n169 = Or(x=w69, y=w13) -> (x .or. y?=w67:bool)
  n170 = And(x=w70, y=w71) -> (x .and. y?=w68:bool)
  n171 = Or(x=w67, y=w68) -> (x .or. y?=w66:bool)
  n172 = Select(t=w1, s=w66, f=0.0) -> (s? t:f=w64:dbl)
  n173 = case shown="False" w151 {
    tunnel: w64 -> [w313 _]
    tunnel: w141 -> [w312 _]
    tunnel: w62 -> [w311 _]
    tunnel: w139 -> [w310 _]
    tunnel: w108 -> [w309 _]
    tunnel: w134 -> [_ w314]
    tunnel: w63 -> [w308 _]
    tunnel: w109 -> [w307 _]
    tunnel: w82 -> [w306 _]
    frame False {
      # "Arm controlled by controller"
      n174 = call <vilib>:"WPI_MotorControlSetOutput.vi"("error in (no error)"=w310, "Output"=w313, "MotorControlDevRef"=w309) -> ()  [unwired: 6 in, 3 out]
      n175 = call <vilib>:"WPI_MotorControlSetOutput.vi"("error in (no error)"=w312, "Output"=w306, "MotorControlDevRef"=w311) -> ()  [unwired: 6 in, 3 out]
      n176 = call <vilib>:"WPI_MotorControlSetOutput.vi"("error in (no error)"=w307, "Output"=w306, "MotorControlDevRef"=w308) -> ()  [unwired: 6 in, 3 out]
    }
    frame True {
      n177 = case shown="4, Default" w314 {
        frame 2 {
          # "X\nPuts arm inside frame"
          n178 = global write "Robot Global Data.vi" "Target Red"(0.0 ("Target Red")) -> ()
          n179 = global write "Robot Global Data.vi" "Target Blue"(0.0 ("Target Blue")) -> ()
        }
        frame 3 {
          # "Y\nPlaces piece on top row"
          n180 = global write "Robot Global Data.vi" "Target Red"(172.089 ("Target Red")) -> ()
          n181 = global write "Robot Global Data.vi" "Target Blue"(54.215 ("Target Blue")) -> ()
        }
        frame 1 {
          # "B\nPlaces piece on middle row"
          n182 = global write "Robot Global Data.vi" "Target Red"(135.831 ("Target Red")) -> ()
          n183 = global write "Robot Global Data.vi" "Target Blue"(19.238 ("Target Blue")) -> ()
        }
        frame 0 {
          # "A\nPlaces piece on bottom row"
          n184 = global write "Robot Global Data.vi" "Target Red"(34.7616 ("Target Red")) -> ()
          n185 = global write "Robot Global Data.vi" "Target Blue"(33.3568 ("Target Blue")) -> ()
        }
        frame 4, Default {
          # "Does not move the arm"
        }
      }
    }
  }
